vi "SubVI_LoopRateDetector.vi"() -> (0 "loop rate (ms)":dbl)   [LabVIEW 2017]
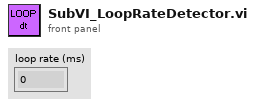
[diagram p1: front panel]
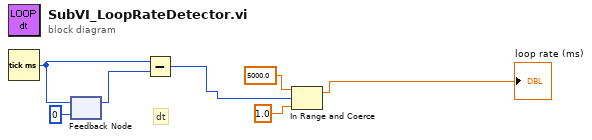
[diagram p0: block diagram]
diagram:
  # "dt"
  n1 = Tick Count (ms)() -> (millisecond timer value=w3:u32)
  n2 = feedback #1(u32 0 ("millisecond timer value")) -> (w4:u32)
  n3 = feedback-in #1(w3) -> ()
  n4 = Subtract(x=w3, y=w4) -> (x-y=w2:u32)
  n5 = In Range and Coerce(upper limit=5000.0, x=w2, lower limit=1.0) -> (coerced(x)=→"loop rate (ms)":dbl)  [unwired: 1 out]
